vi "twm_dmm_open.vi"(9 "ssn":u8[](array[numeric]), 10 "dmm visa":string[](array[string])) -> (0 "error out":errorcluster, 1 "sync unit idn string":string, 2 "awg idn string":string, 3 "dmm(s) idn strings":string[](array[string]), 4 "ssn out":u8[](array[numeric]))   [LabVIEW 2013, in "3458A Virtual Digitizer.lvlib"]
uses:
  3458A Virtual Digitizer.lvlib
  3458A Digitizer Session.ctl
  3458A Virtual Channel Config.ctl
  Counter/Counter Session.ctl
  Counter/Counter Type.ctl
  AWG/AWG Session.ctl
  AWG/AWG Type.ctl
  3458A Sync Mode.ctl
  3458A Idn Mode.ctl
  3458A Digitizing Low Levels/Configure/Sampling Mode.ctl
  3458A Digitizing Process Options.ctl
  3458A Data Packet.ctl
  3458A Aux Record Data.ctl
  3458A Digitizing Low Levels/Configure/Level Setup.ctl
  3458A Digitizing Low Levels/Configure/First Sample Trigger.ctl
  Counter/Counter.lvlib
  AWG/AWG.lvlib
  3458A Digitizing Low Levels/3458A Digitizing Low Levels.lvlib
panel:
  in  "Range [Vpk]":dbl format="%#_13g"
  in  "reset instruments (False)":bool
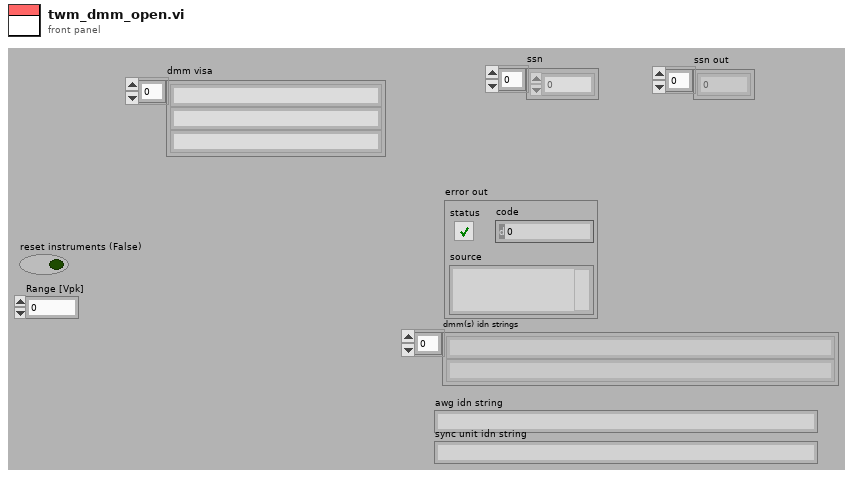
[diagram p1: front panel]
types:
  T1 = typedef "3458A Virtual Digitizer.lvlib/3458A Digitizer Session.ctl" = cluster{"channels":T2[], "sync unit":T3, "awg unit":T5, "sync mode":T7, "streaming mode":bool, "idn mode":T8, "sampling mode":T9, "Ts [s]":dbl, "sample memory [B]":i32, "proc setup":T10, "sample size [B]":i32, "sample count":i32, "aux data":T12, "ranges [V]":dbl[], "aperture [s]":dbl, "LEVEL trigger":T13, "trigger mode":T14, "measure temp.?":bool, "disp mesages":string[], "shared bus?":bool}
  T2 = typedef "3458A Virtual Digitizer.lvlib/3458A Virtual Channel Config.ctl" = cluster{"VISA":refnum<visa-resource-name>, "Range [Vpk]":dbl}
  T3 = typedef "Counter.lvlib/Counter Session.ctl" = cluster{"VISA":refnum<visa-resource-name>, "type":T4}
  T4 = typedef "Counter.lvlib/Counter Type.ctl" = enum16{"Picotest U6200A", "dummy"}
  T5 = typedef "AWG.lvlib/AWG Session.ctl" = cluster{"type":T6, "VISA":refnum<visa-resource-name>, "enable 10MHz ref":bool}
  T6 = typedef "AWG.lvlib/AWG Type.ctl" = enum16{"Agilent 331xxA to 332xxA", "Agilent 335xxA to 336xxA", "dummy"}
  T7 = typedef "3458A Virtual Digitizer.lvlib/3458A Sync Mode.ctl" = enum16{"MASTER-SLAVE, MASTER clocked by TIMER", "MASTER-SLAVE, MASTER clocked by AWG", "ALL clocked by AWG", "MASTER-SLAVE, ALL clocked by TIMER", "ALL clocked by AWG with DFLL"}
  T8 = typedef "3458A Virtual Digitizer.lvlib/3458A Idn Mode.ctl" = enum16{"Auto", "Sequential (chn A, chn B, ...)", "From calibration string"}
  T9 = typedef "3458A Virtual Digitizer.lvlib/3458A Digitizing Low Levels.lvlib/Sampling Mode.ctl" = enum16{"DCV", "DSDC", "DSAC"}
  T10 = typedef "3458A Virtual Digitizer.lvlib/3458A Digitizing Process Options.ctl" = cluster{"channel id":i32, "packet size [smpl]":i32, "current timeout [s]":dbl, "blk2blk timeout [s]":dbl, "event time":timestamp, "stop notifier":refnum<notifier>, "data queues":refnum<queue>[], "proc refs":refnum<vi>[], "bus semaphore":T11}
  T11 = typedef "Semaphore RefNum" = refnum<k1>
  T12 = typedef "3458A Virtual Digitizer.lvlib/3458A Aux Record Data.ctl" = cluster{"channel id":i32, "valid?":bool[], "gain [V]":dbl[], "timestamp [s]":dbl[], "Ts [s]":dbl, "abs timestamp":timestamp, "t [deg C]":dbl[]}
  T13 = typedef "3458A Virtual Digitizer.lvlib/3458A Digitizing Low Levels.lvlib/Level Setup.ctl" = cluster{"edge":enum16{"POS", "NEG"}, "level [V]":dbl, "coupling":enum16{"DC", "AC"}}
  T14 = typedef "3458A Virtual Digitizer.lvlib/3458A Digitizing Low Levels.lvlib/First Sample Trigger.ctl" = enum16{"AUTO", "EXT", "SYN", "SGL", "HOLD", "LEVEL"}
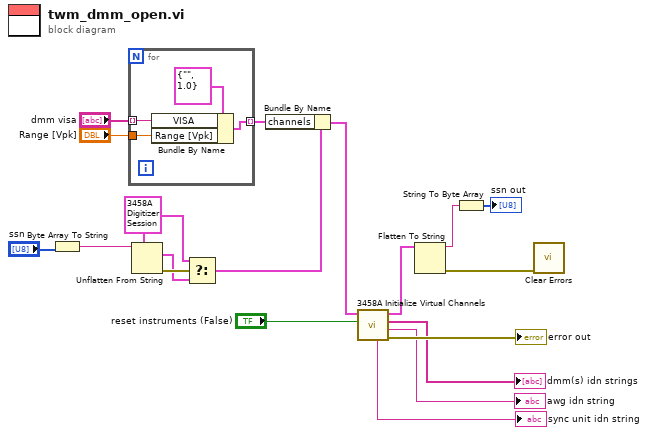
[diagram p0: block diagram]
diagram:
  w8 = T1 {"channels"=[{"VISA"="GPIB1::22::INSTR", "Range [Vpk]"=10.0}, {"VISA"="GPIB1::16::INSTR", "Range [Vpk]"=1.0}], "sync unit"={"VISA"="", "type"=enum."Picotest U6200A"}, "awg unit"={"type"=enum."Agilent 331xxA to 332xxA", "VISA"="", "enable 10MHz ref"=FALSE}, "sync mode"=enum."MASTER-SLAVE, MASTER clocked by TIMER", "streaming mode"=FALSE, "idn mode"=enum."Auto", "sampling mode"=enum."DCV", "Ts [s]"=0.0002, "sample memory [B]"=20480, "proc setup"={"channel id"=0, "packet size [smpl]"=250, "current timeout [s]"=10.0, "blk2blk timeout [s]"=10.0, "event time"=timestamp(0 s since 1904-01-01), "stop notifier"=refnum, "data queues"=[refnum, refnum], "proc refs"=[refnum, refnum], "bus semaphore"=refnum}, "sample size [B]"=4, "sample count"=1000, "aux data"={"channel id"=0, "valid?"=[TRUE, TRUE], "gain [V]"=[1.18824752e-05, 1.19876853e-06], "timestamp [s]"=[0.0, 0.0], "Ts [s]"=0.0002, "abs timestamp"=timestamp(0 s since 1904-01-01), "t [deg C]"=[nan, nan]}, "ranges [V]"=[10.0, 1.0], "aperture [s]"=5e-05, "LEVEL trigger"={"edge"=enum."POS", "level [V]"=0.0, "coupling"=enum."DC"}, "trigger mode"=enum."AUTO", "measure temp.?"=FALSE, "disp mesages"=["CHN-1", "CHN-2"], "shared bus?"=TRUE} ("session")
  n1 = Byte Array To String(unsigned byte array="ssn") -> (string=w3:string)
  n2 = for {
    tunnel: "dmm visa" -> [w21] mode=indexing
    tunnel: [w23] -> w12 mode=indexing
    tunnel: "Range [Vpk]" -> [w20]
    n3 = Bundle By Name(cluster=T2 {"VISA"="", "Range [Vpk]"=1.0} ("dmm channel"), "VISA"=w21, "Range [Vpk]"=w20) -> (w23:T2)
  }
  n4 = Unflatten From String(type=w8, binary string=w3) -> (value=w7:T1, error out=w9:errorcluster)  [unwired: 3 in, 1 out]
  n5 = Select(t=w8, s=w9, f=w7) -> (s? t:f=w6:T1)
  n6 = Bundle By Name(cluster=w6, "channels"=w12) -> (w18:T1)
  n7 = call "3458A Initialize Virtual Channels.vi"("reset instruments (False)"="reset instruments (False)", "digitizer in"=w18) -> ("error out"=→"error out":errorcluster, "awg idn string"=→"awg idn string":string, "dmm(s) idn strings"=→"dmm(s) idn strings":string[], "digitizer out"=w10:T1, "sync unit idn string"=→"sync unit idn string":string)  [unwired: 5 in]
  n8 = Flatten To String(anything=w10) -> (data string=w2:string, error out=w5:errorcluster)  [unwired: 3 in, 1 out]
  n9 = String To Byte Array(string=w2) -> (unsigned byte array=→"ssn out":u8[])
  n10 = call <vilib>:"Clear Errors.vi"("error in (no error)"=w5) -> ()  [unwired: 6 in, 1 out]
